vi "TestDll.vi"() -> ()   [LabVIEW 2017]
uses:
  D:/Project/Tymphany/LT_UpgradeFlash/New_Lib/LT_UpgradeFlash_dll/LT_UpgradeFlash_dll/bin/Debug/LT_UpgradeFlash_dll.dll
  LT_UpgradeFlash_dll/LT_UpgradeFlash_dll/bin/Debug/LT_UpgradeFlash_dll.dll
panel:
  in  "progFilePath":path=path "D:/Project/Tymphany/LT_UpgradeFlash/HDMI Board/LT FW  Files/LT9611 UXC/lt9611uxc_fw.bin"
  out "resultStr":string
  out "Prog":bool
  in  "Prog_btn":bool
  out "SelectChip":bool
  in  "chipName_en":u16(ring) items=["LT6911", "LT9611"]
  in  "selectChip_btn":bool
  out "resultString":string
  out "Erase":bool
  in  "Erase_btn":bool
  in  "read_btn":bool
  in  "open exe btn":bool
  in  "Stop_btn":bool
  out "resultString":string
  out "ClickReadButton":bool
  out "OpenExeOK":bool
  in  "exePath":path=path "D:/Project/Tymphany/LT_UpgradeFlash/HDMI Board/LT Upgrade Flash/Upgrade_Flash_For_Application.exe"
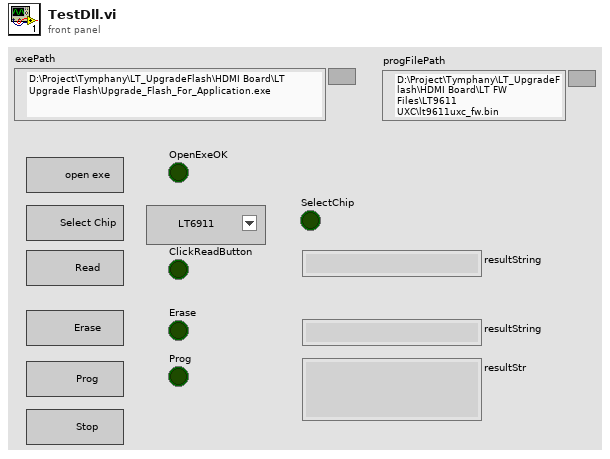
[diagram p1: front panel]
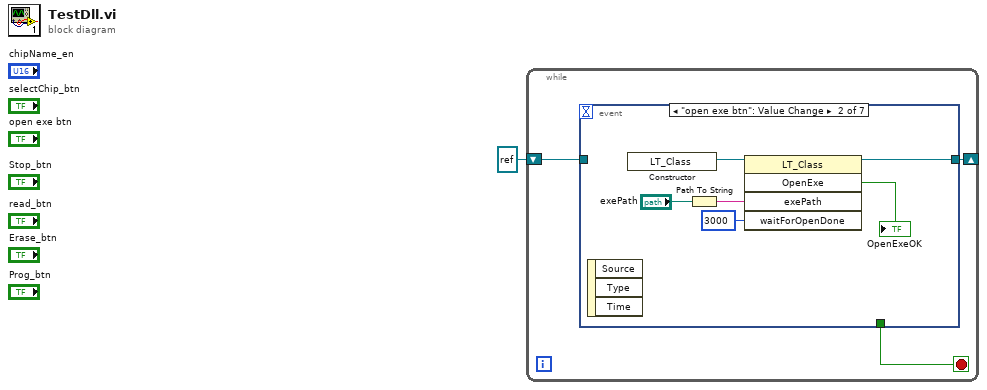
[diagram p0: block diagram]
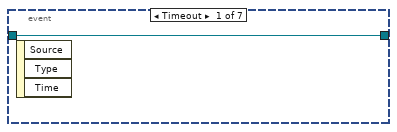
[diagram p2: hidden frame]
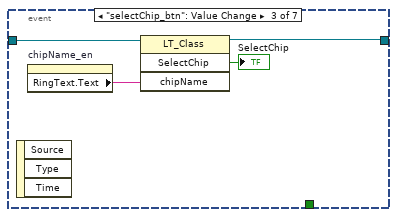
[diagram p3: hidden frame]
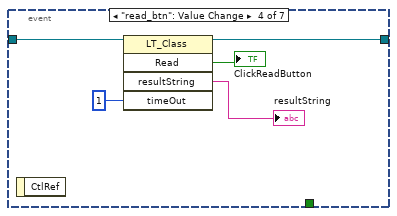
[diagram p4: hidden frame]
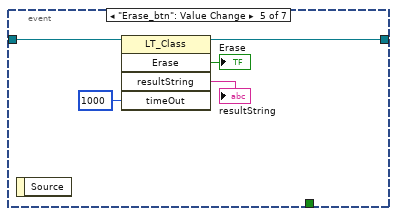
[diagram p5: hidden frame]
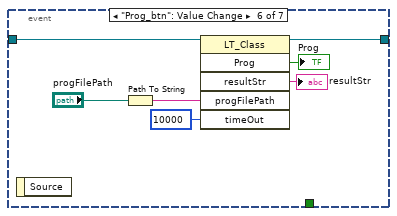
[diagram p6: hidden frame]
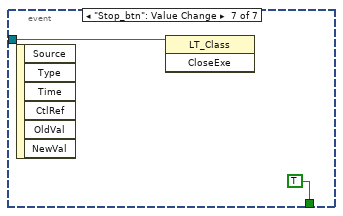
[diagram p7: hidden frame]
diagram:
  n1 = while {
    shift-right: [w3] -> _
    shift-left: refnum<k24> refnum ("new reference") -> [w2]
    stop <- w4 stop-if-true
    n2 = event shown="[1] \"open exe btn\": Value Change" {
      selector: _ -> [_ _ _ _ _ _ _]
      dyn-events: _ -> [_ _ _ _ _ _ _]
      timeout: _ -> [_ _ _ _ _ _ _]
      tunnel: [_ _ _ _ _ _ TRUE] -> w4
      tunnel: [w5 w6 w14 w16 w24 w31 _] -> w3
      tunnel: w2 -> [w5 _ w15 w20 w25 w32 w33]
      event Timeout {
        n3 = event-data() -> ()  [unwired: 1 in, 3 out]
      }
      event "open exe btn": Value Change {
        n4 = event-data() -> ()  [unwired: 1 in, 3 out]
        n5 = constructor class="LT_Class"() -> (reference out=w9:refnum<k24>)  [unwired: 3 in, 2 out]
        n6 = Path To String(path="exePath") -> (string=w10:string)
        n7 = invoke class="LT_Class" method="OpenExe"(reference=w9, "exePath"=w10, "waitForOpenDone"=3000) -> (reference out=w6:refnum<k24>, "OpenExe"=→"OpenExeOK":bool)  [unwired: 2 in, 3 out]
      }
      event "selectChip_btn": Value Change {
        n8 = event-data() -> ()  [unwired: 1 in, 3 out]
        n9 = property on="chipName_en" class="Ring (strict)"() -> ("RingText.Text"=w13:string)  [unwired: 2 in, 2 out]
        n10 = invoke class="LT_Class" method="SelectChip"(reference=w15, "chipName"=w13) -> (reference out=w14:refnum<k24>, "SelectChip"=→"SelectChip":bool)  [unwired: 2 in, 2 out]
      }
      event "read_btn": Value Change {
        n11 = event-data() -> ()  [unwired: 1 in, 1 out]
        n12 = invoke class="LT_Class" method="Read"(reference=w20, "timeOut"=1) -> (reference out=w16:refnum<k24>, "Read"=→"ClickReadButton":bool, "resultString"=→"resultString":string)  [unwired: 3 in, 2 out]
      }
      event "Erase_btn": Value Change {
        n13 = event-data() -> ()  [unwired: 1 in, 1 out]
        n14 = invoke class="LT_Class" method="Erase"(reference=w25, "timeOut"=1000) -> (reference out=w24:refnum<k24>, "Erase"=→"Erase":bool, "resultString"=→"resultString":string)  [unwired: 3 in, 2 out]
      }
      event "Prog_btn": Value Change {
        n15 = event-data() -> ()  [unwired: 1 in, 1 out]
        n16 = Path To String(path="progFilePath") -> (string=w26:string)
        n17 = invoke class="LT_Class" method="Prog"(reference=w32, "progFilePath"=w26, "timeOut"=10000) -> (reference out=w31:refnum<k24>, "Prog"=→"Prog":bool, "resultStr"=→"resultStr":string)  [unwired: 3 in, 3 out]
      }
      event "Stop_btn": Value Change {
        n18 = event-data() -> ()  [unwired: 1 in, 6 out]
        n19 = invoke class="LT_Class" method="CloseExe"(reference=w33) -> ()  [unwired: 2 in, 3 out]
      }
    }
  }
